vi "MUX80_Split_Page_String.vi"(0 "Array In":string[](array[string])) -> (1 "Page 1 out":string[](array[string]), 2 "Page 6 out":string[](array[string]), 3 "Page 2 out":string[](array[string]), 4 "Page 3 out":string[](array[string]), 5 "Page 4 out":string[](array[string]), 6 "Page 5 out":string[](array[string]))   [LabVIEW 2020]
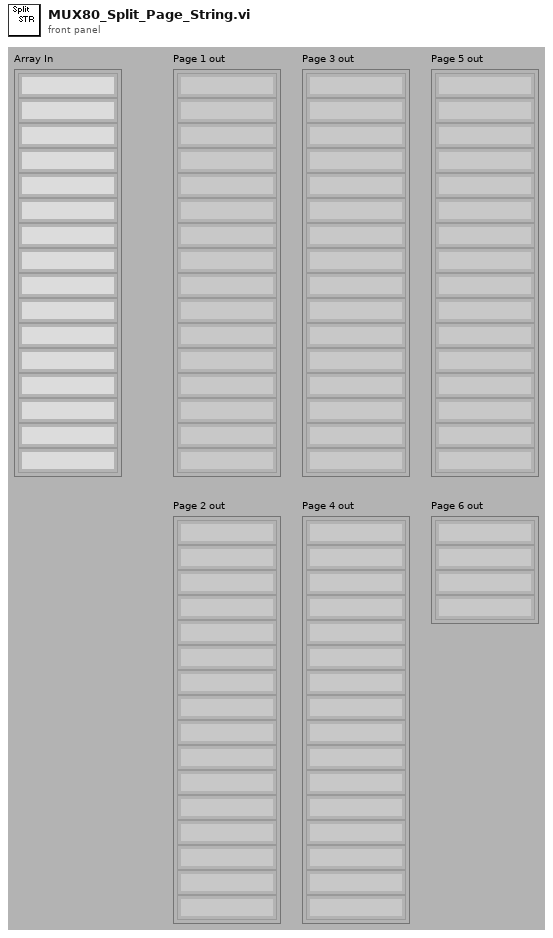
[diagram p1: front panel]
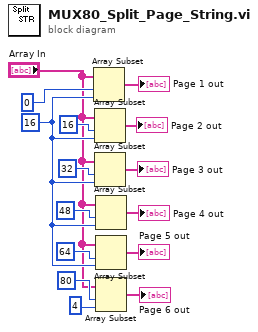
[diagram p0: block diagram]
diagram:
  w9 = 16
  n1 = Array Subset(array="Array In", index=0, length=w9) -> (→"Page 1 out":string[])
  n2 = Array Subset(array="Array In", index=16, length=w9) -> (→"Page 2 out":string[])
  n3 = Array Subset(array="Array In", index=32, length=w9) -> (→"Page 3 out":string[])
  n4 = Array Subset(array="Array In", index=48, length=w9) -> (→"Page 4 out":string[])
  n5 = Array Subset(array="Array In", index=64, length=w9) -> (→"Page 5 out":string[])
  n6 = Array Subset(array="Array In", index=80, length=4) -> (→"Page 6 out":string[])
